vi "Export Final Data.vi"(8 "error in (no error)":errorcluster, 11 "Scan Data Process in":T1) -> (0 "error out":errorcluster, 3 "Scan Data Process out":T1)   [LabVIEW 2015, in "Exposure Process.lvlib"]
uses:
  Exposure Process.lvlib
  Control_Scan Data Process.ctl
  <vilib>/addons/PointValueMap/controls/PointMap.ctl
  Control_EXP Information.ctl
  Control_File Save Setup.ctl
  Control_Enable and Path.ctl
  Control_ICM Export Setting.ctl
  <vilib>/addons/PointValueMap/PointValueMap.lvlib
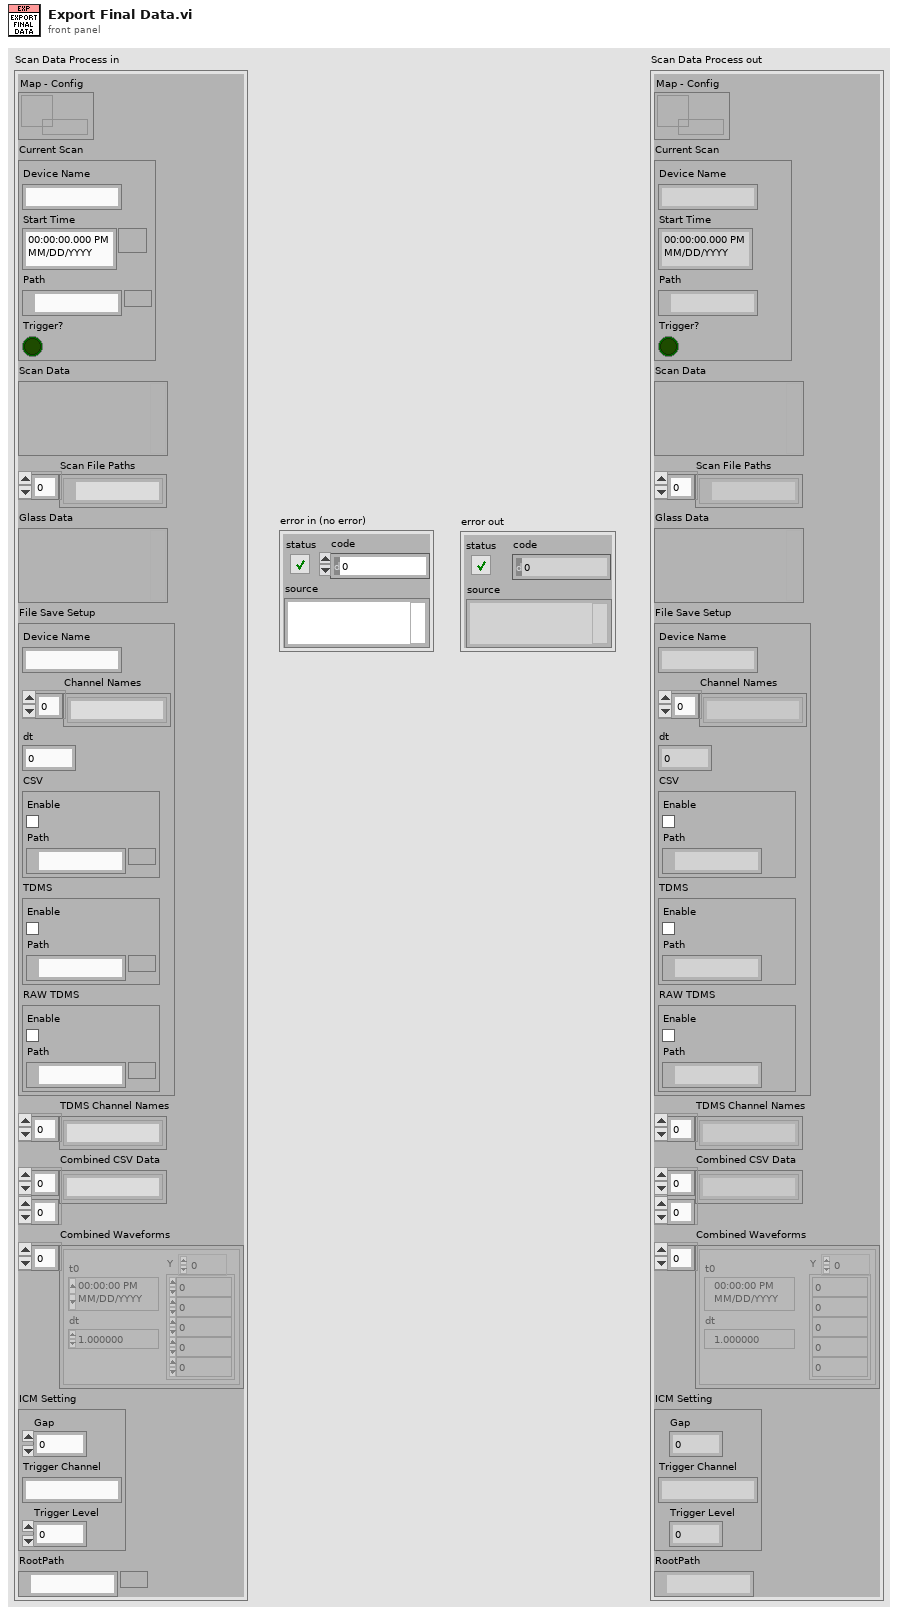
[diagram p1: front panel]
types:
  T1 = typedef "Exposure Process.lvlib/Control_Scan Data Process.ctl" = cluster{"Map - Config":T2, "Current Scan":T3, "Scan Data":variant, "Scan File Paths":path[], "Glass Data":variant, "File Save Setup":T4, "TDMS Channel Names":string[], "Combined CSV Data":string[][], "Combined Waveforms":waveform(dbl)[], "ICM Setting":T6, "RootPath":path}
  T2 = typedef "PointValueMap.lvlib/PointMap.ctl" = refnum<data-value>
  T3 = typedef "Exposure Process.lvlib/Control_EXP Information.ctl" = cluster{"Device Name":string, "Start Time":timestamp, "Path":path, "Trigger?":bool}
  T4 = typedef "Exposure Process.lvlib/Control_File Save Setup.ctl" = cluster{"Device Name":string, "Channel Names":string[], "dt":dbl, "CSV":T5, "TDMS":T5, "RAW TDMS":T5}
  T5 = typedef "Exposure Process.lvlib/Control_Enable and Path.ctl" = cluster{"Enable":bool, "Path":path}
  T6 = typedef "Exposure Process.lvlib/Control_ICM Export Setting.ctl" = cluster{"Gap":dbl, "Trigger Channel":string, "Trigger Level":dbl}
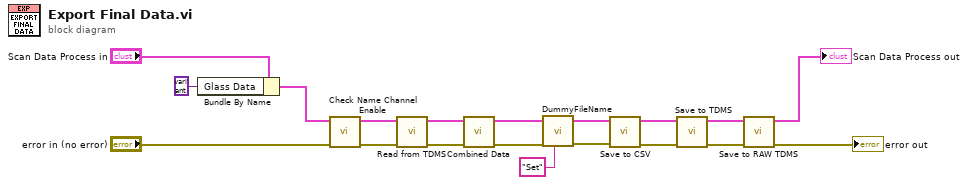
[diagram p0: block diagram]
diagram:
  n1 = Bundle By Name(cluster="Scan Data Process in", "Glass Data"=variant) -> (w16:T1)
  n2 = call "Check Name Channel Enable.vi"("error in (no error)"="error in (no error)", "Scan Data Process in"=w16) -> ("error out"=w15:errorcluster, "Scan Data Process out"=w14:T1)  [unwired: 8 in]
  n3 = call "Read from TDMS.vi"("error in (no error)"=w15, "Scan Data Process in"=w14) -> ("error out"=w12:errorcluster, "Scan Data Process out"=w13:T1)  [unwired: 8 in]
  n4 = call "Combined Data.vi"("error in (no error)"=w12, "Scan Data Process in"=w13) -> ("error out"=w3:errorcluster, "Scan Data Process out"=w11:T1)  [unwired: 8 in]
  n5 = call "DummyFileName.vi"("Function"="Set", "error in (no error)"=w3) -> ("error out"=w2:errorcluster)  [unwired: 8 in, 1 out]
  n6 = call "Save to CSV.vi"("error in (no error)"=w2, "Scan Data Process"=w11) -> ("error out"=w9:errorcluster, "Scan Data Process out"=w10:T1)  [unwired: 8 in]
  n7 = call "Save to TDMS.vi"("error in (no error)"=w9, "Scan Data Process in"=w10) -> ("error out"=w7:errorcluster, "Scan Data Process out"=w8:T1)  [unwired: 8 in]
  n8 = call "Save to RAW TDMS.vi"("error in (no error)"=w7, "Scan Data Process"=w8) -> ("error out"=→"error out":errorcluster, "Scan Data Process out"=→"Scan Data Process out":T1)  [unwired: 8 in]
